vi "crosscor_sub1.vi"(0 "Array 3":i32[](array[numeric]), 1 "router channels":u8[](array[numeric]), 2 "macro times":u32[](array[numeric]), 3 "Array 2":i32[](array[numeric]), 4 "Numerisch 2":u8, 5 "Numerisch":u8, 8 "Boolesch":bool) -> (6 "macro times 2":u32[](array[numeric]), 7 "macro times 3":u32[](array[numeric]))   [LabVIEW 2009]
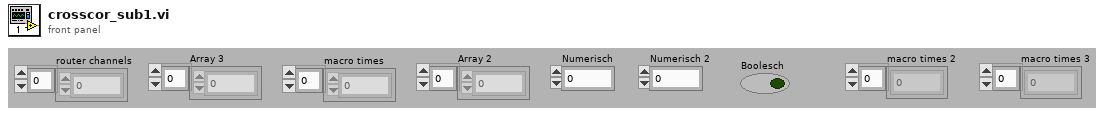
[diagram p1: front panel]
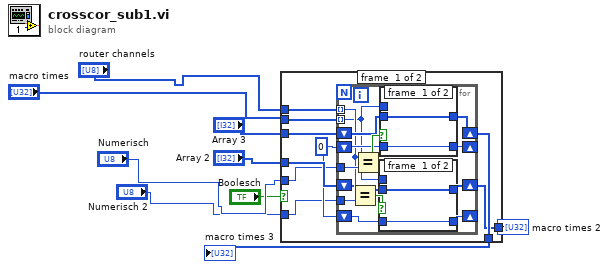
[diagram p0: block diagram]
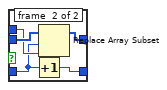
[diagram p2: hidden frame]
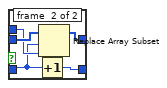
[diagram p3: hidden frame]
diagram:
  n1 = case shown="False" "Boolesch" {
    tunnel: "macro times" -> [w18 w47]
    tunnel: "Array 3" -> [w17 _]
    tunnel: "Numerisch" -> [w10 _]
    tunnel: "router channels" -> [w16 _]
    tunnel: [w15 w47] -> w3
    tunnel: "Numerisch 2" -> [w11 _]
    tunnel: "Array 2" -> [w14 _]
    tunnel: [w12 w47] -> w5
    frame #0 {
      w13 = u32 0 ("element")
      n2 = for {
        tunnel: w18 -> [w23] mode=indexing
        shift-right: [w29] -> w15
        shift-left: w17 -> [w30]
        tunnel: w10 -> [w31]
        tunnel: w16 -> [w26] mode=indexing
        shift-right: [w27] -> _
        shift-left: w13 -> [w28]
        tunnel: w11 -> [w25]
        shift-right: [w20] -> w12
        shift-left: w14 -> [w22]
        shift-right: [w19] -> _
        shift-left: w13 -> [w21]
        n3 = Equal?(x=w26, y=w25) -> (x = y?=w24:bool)
        n4 = Equal?(x=w26, y=w31) -> (x = y?=w32:bool)
        n5 = case shown="True" w24 {
          tunnel: w22 -> [w34 w39]
          tunnel: [w34 w38] -> w20
          tunnel: w23 -> [_ w37]
          tunnel: w21 -> [w33 w35]
          tunnel: [w33 w36] -> w19
          frame #0 {
          }
          frame #1 {
            n6 = Increment(x=w35) -> (x+1=w36:u32)
            n7 = Replace Array Subset(array=w39, new element=w37, index=w35) -> (w38:i32[])
          }
        }
        n8 = case shown="True" w32 {
          tunnel: w30 -> [w41 w46]
          tunnel: [w41 w45] -> w29
          tunnel: w23 -> [_ w44]
          tunnel: w28 -> [w40 w42]
          tunnel: [w40 w43] -> w27
          frame #0 {
          }
          frame #1 {
            n9 = Increment(x=w42) -> (x+1=w43:u32)
            n10 = Replace Array Subset(array=w46, new element=w44, index=w42) -> (w45:i32[])
          }
        }
      }
    }
    frame #1 {
    }
  }
  "macro times 2" <- w5
  "macro times 3" <- w3
